vi "initialise.vi"(8 "error in (no error)":errorcluster, 11 "SignalReaderCN091129DAQmx in":refnum<class "SignalReaderCN091129DAQmx.lvclass">) -> (0 "error out":errorcluster, 3 "SignalReaderCN091129DAQmx out":refnum<class "SignalReaderCN091129DAQmx.lvclass">)   [LabVIEW 2010, in "SignalReaderCN091129DAQmx.lvclass"]
doc: "The dynamic dispatch-version of this VI initalises the plug-in object by allocating and initalising any dynamic resources need."
uses:
  SignalReaderCN091129DAQmx.lvclass
  GenericSignalReader/GenericSignalReader/GenericSignalReader.lvclass
  SignalReaderCN091129DAQmx.lvclass/SignalReaderCN091129DAQmx.ctl
  <vilib>/DAQmx/create/channels.llb/DAQmx Create Channel (AI-Voltage-Basic).vi
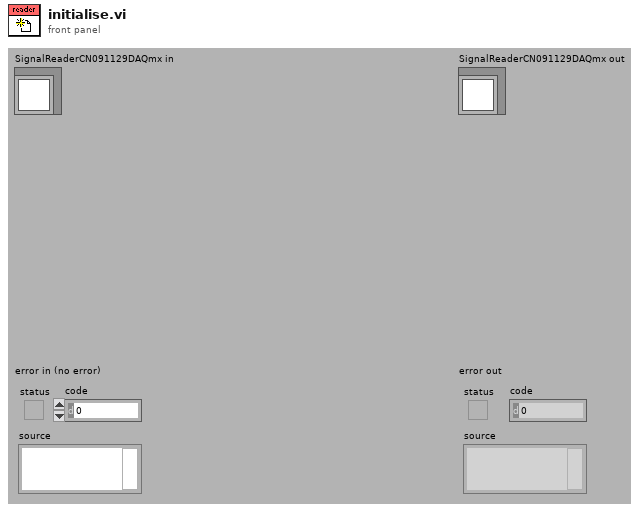
[diagram p1: front panel]
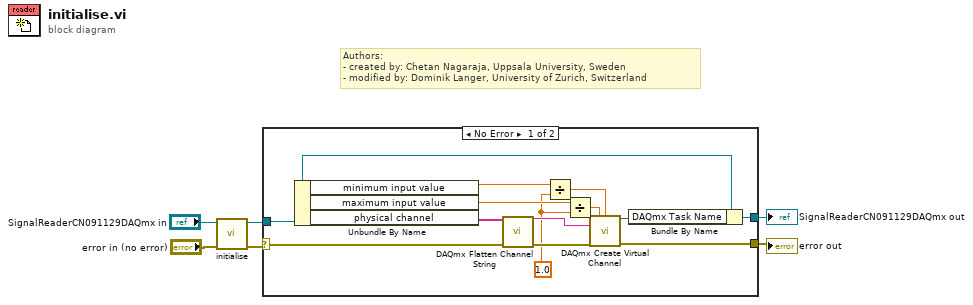
[diagram p0: block diagram]
diagram:
  # "Authors: \n- created by: Chetan Nagaraja, Uppsala University, Sweden\n- modified by: Dominik Langer, University of Zurich, Switzerland"
  n1 = call-parent "initialise.vi"("error in (no error)"="error in (no error)", "GenericPlugin in"="SignalReaderCN091129DAQmx in") -> ("error out"=w4:errorcluster, "GenericPlugin out"=w2:refnum<class "SignalReaderCN091129DAQmx.lvclass">)  [unwired: 8 in]
  n2 = case shown="No Error" w4 {
    selector: w4 -> [w18 w21]
    tunnel: [w8 w21] -> w3
    tunnel: w2 -> [w10 w20]
    tunnel: [w9 w20] -> w1
    frame No Error {
      w13 = dbl[unit] 1.0 ("y")
      n3 = Unbundle By Name(w10) -> ("minimum input value"=w15:dbl[unit], "maximum input value"=w14:dbl[unit], "physical channel"=w19:string[])
      n4 = call <vilib>:"DAQmx Flatten Channel String.vi"("names in"=w19, "error in"=w18) -> ("names out"=w16:string, "error out"=w17:errorcluster)  [unwired: 12 in]
      n5 = Divide(x=w15, y=w13) -> (x/y=w12:dbl)
      n6 = Divide(x=w14, y=w13) -> (x/y=w11:dbl)
      n7 = call-poly <vilib>:"DAQmx Create Virtual Channel.vi"("maximum value"=w11, "minimum value"=w12, "physical channels"=w16, "error in"=w17) -> ("task out"=w7:refnum<k21>, "error out"=w8:errorcluster)  [unwired: 10 in]
      n8 = Bundle By Name(cluster=w10, "DAQmx Task Name"=w7) -> (w9:refnum<class "SignalReaderCN091129DAQmx.lvclass">)
    }
    frame Error {
    }
  }
  "error out" <- w3
  "SignalReaderCN091129DAQmx out" <- w1
